vi "Set On-Line Status.vi"(8 "error in (no error)":errorcluster, 10 "On-Line":bool, 11 "Scenarios Class in":refnum<class "Scenarios Class.lvclass">) -> (0 "error out":errorcluster, 3 "Scenarios Class out":refnum<class "Scenarios Class.lvclass">)   [LabVIEW 2020, in "SECS Scenarios.lvlib" / "Scenarios Class.lvclass"]
uses:
  Scenarios Class.lvclass
  Scenarios Class.lvclass/Scenarios Class.ctl
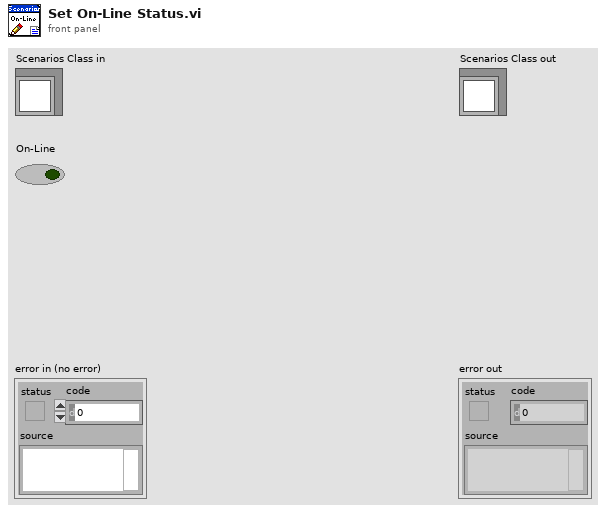
[diagram p1: front panel]
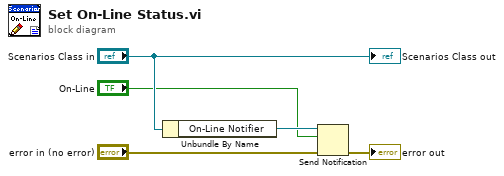
[diagram p0: block diagram]
diagram:
  n1 = Unbundle By Name("Scenarios Class in") -> ("On-Line Notifier"=w3:refnum<notifier>)
  n2 = Send Notification(notification="On-Line", notifier=w3, error in (no error)="error in (no error)") -> (error out=→"error out":errorcluster)  [unwired: 1 out]
  "Scenarios Class out" <- "Scenarios Class in"
